vi "main.vi"() -> ()   [LabVIEW 2014]
uses:
  <vilib>/picture/3D Picture Control/Object/Create Object (drawable).vi
  <vilib>/picture/3D Picture Control/Object/Add Object (reference).vi
  <vilib>/Instr/_visa.llb/VISA Configure Serial Port (Instr).vi
  <vilib>/picture/3D Picture Control/NI_3D Picture Control.lvlib
panel:
  out "长度（剩余）":u8
  out "?":u8[](array[numeric])
  in  "选项卡控件":T1
  in  "?":bool
  in  "D":i16
  in  "P":i16
  in  "I":i16
  out "布尔":bool
  out "AcceZ":i32
  out "AcceY":i32
  out "加速度":cluster{dbl, dbl, dbl}(graph)
  out "AcceX":i32
  out "HEANDING":i32
  out "BANK":i32
  out "模块4 2":bool
  out "模块3 2":bool
  out "模块2 2":bool
  out "模块1 2":bool
  out "模块4":bool
  out "模块3":bool
  out "模块2":bool
  out "模块1":bool
  out "PITCH":i32
  in  "停止":bool
  in  "打开":bool caption="stop"
  in  "校验位：":u16(ring) items=["  无校验", "  奇校验", "  偶校验"]
  in  "波特率：":u16(ring)=11 items=["   300", "   600", "   1200", "   2400", "   4800   ", "   9600", "   19200", "   38400", "   43000", "   56000", "   57600", "   115200"]
  in  "通讯口：":u16(ring) items=["   com1", "   com2", "   com3", "   com4", "   com5"]
  out "姿态":cluster{dbl, dbl, dbl}(graph) caption="波形图表"
  in  "上下移动":dbl(slide) scale=-10.0..10.0
  in  "左右移动":dbl(slide) scale=-10.0..10.0
  in  "前后移动":dbl(slide) scale=-10.0..10.0
  in  "缩放":dbl(knob)=2.2771854734286614 scale=0.0..10.0
  out "三维图片":refnum<vi>(3d-picture)
  out "工作指示灯":bool
  # "EVA-MPU6050姿态测试平台"
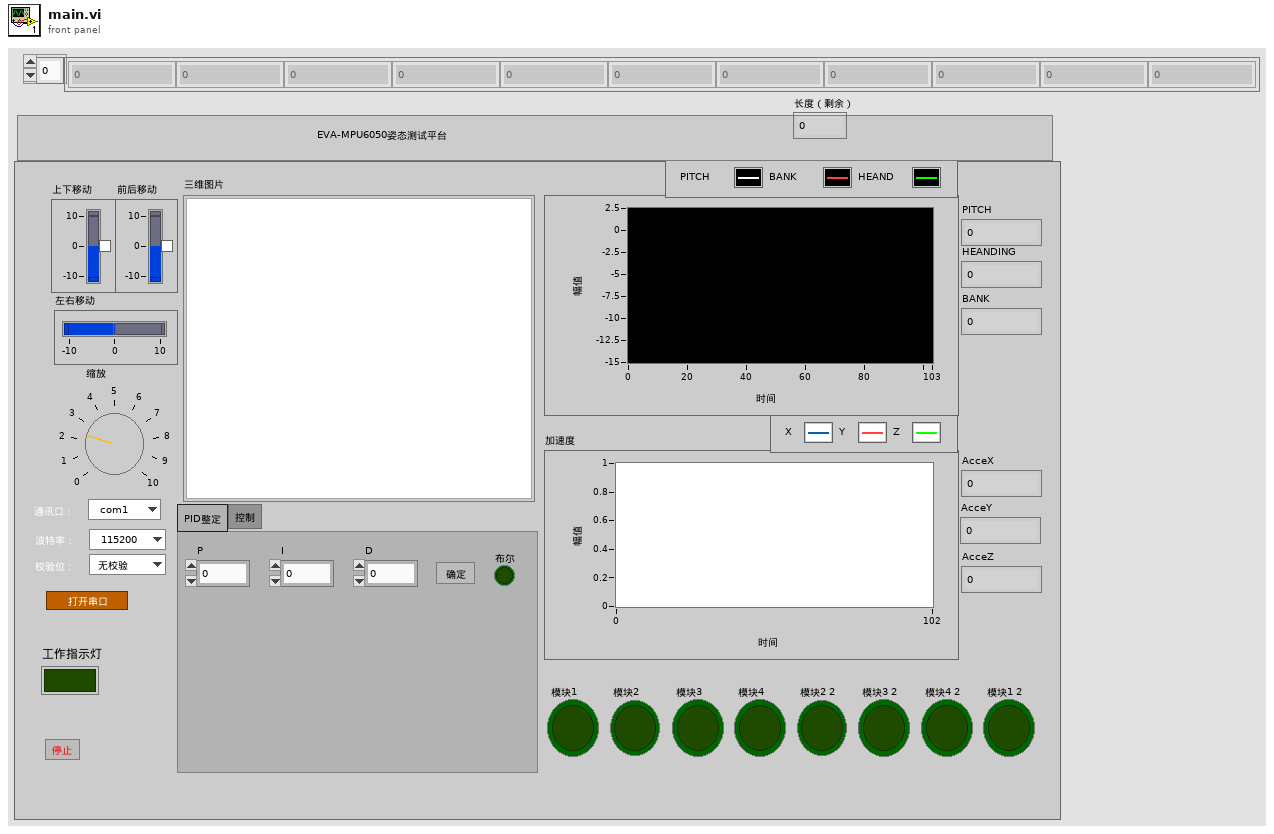
[diagram p1: front panel]
types:
  T1 = typedef "选项卡1.ctl" = enum32{"PID整定", "控制"}
  T2 = cluster{"PITCH":i32, "BANK":i32, "HEANDING":i32, "X":i32, "Y":i32, "Z":i32}
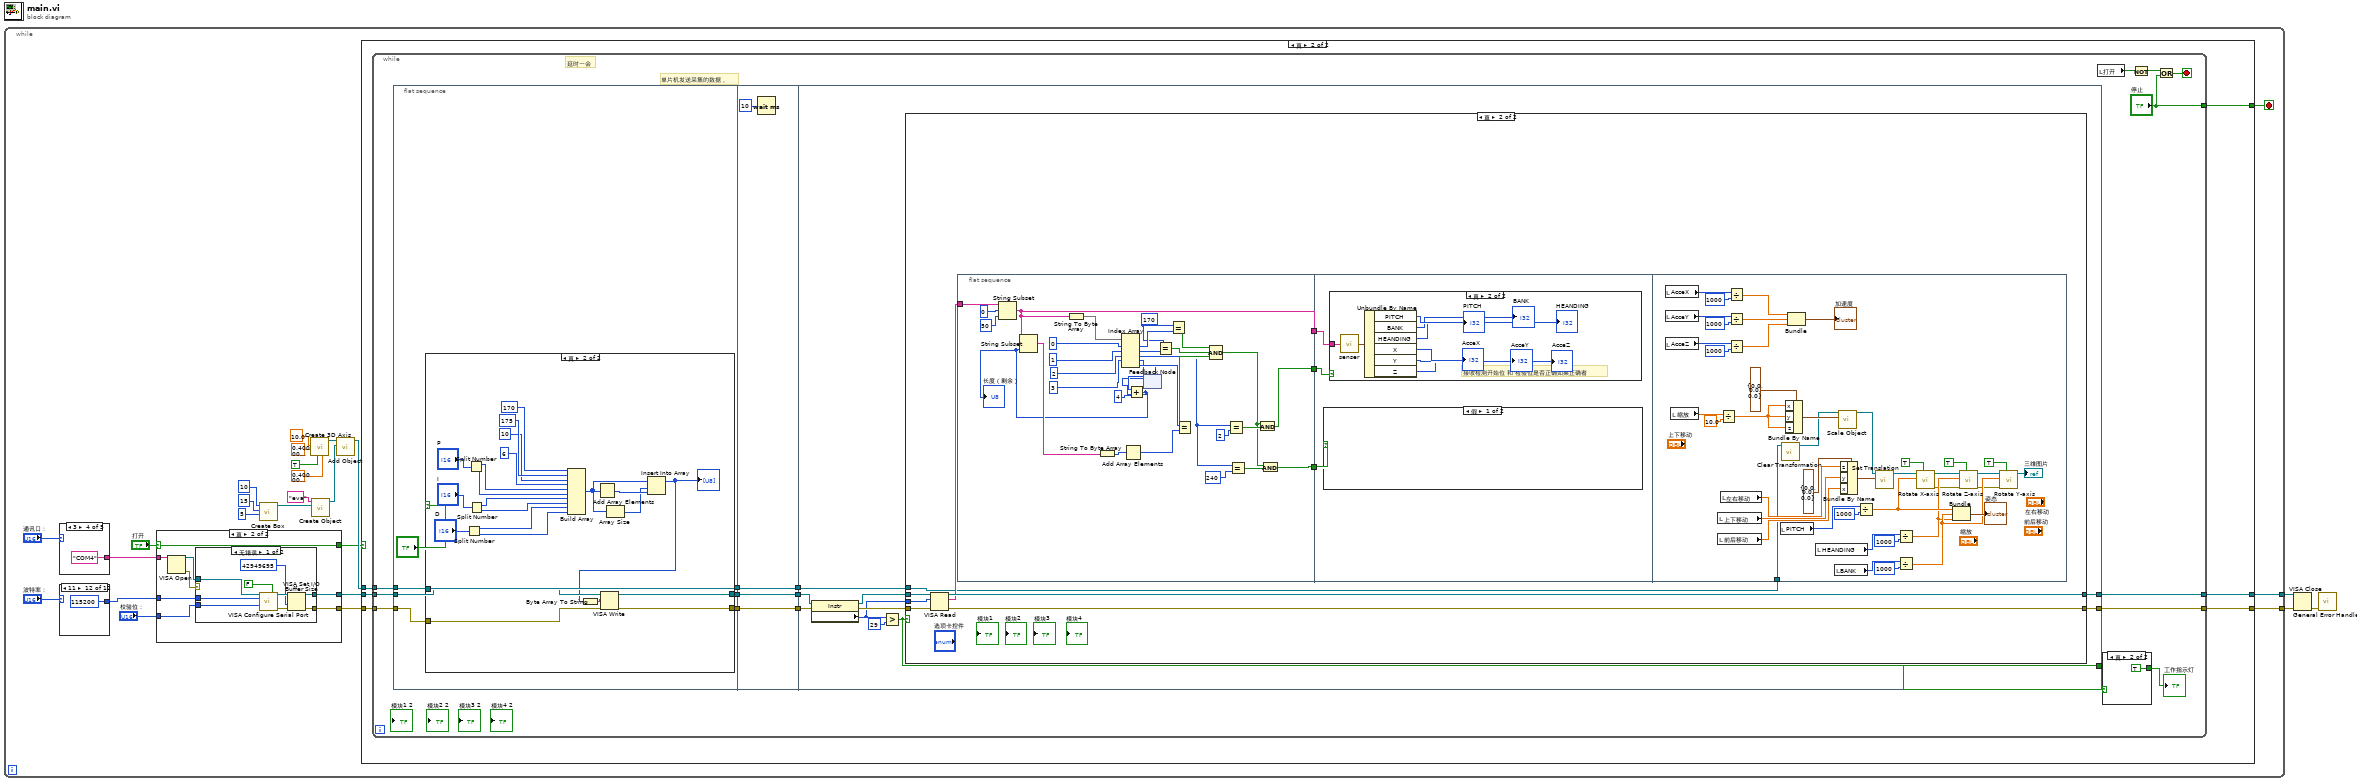
[diagram p0: block diagram]
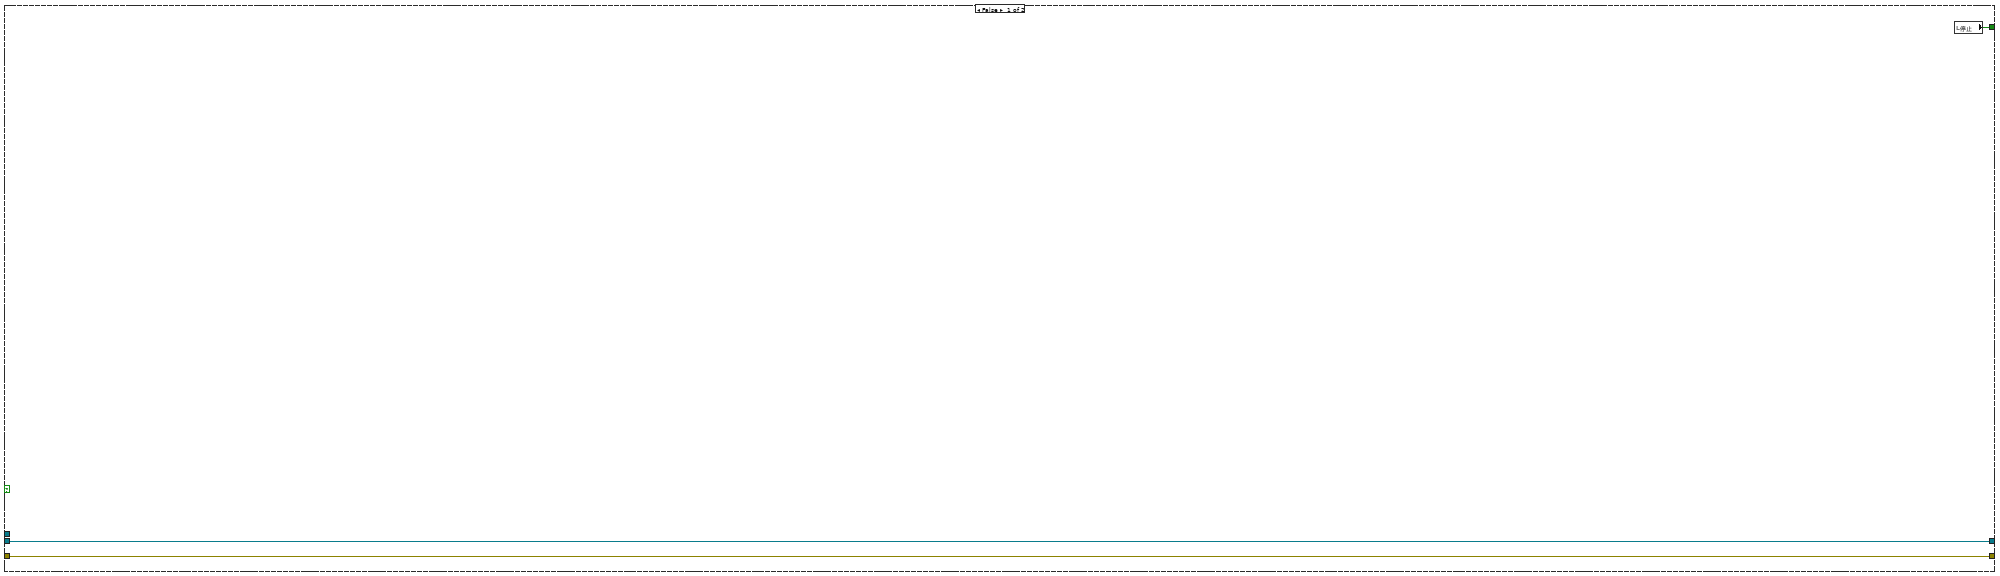
[diagram p2: hidden frame]
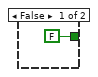
[diagram p3: hidden frame]
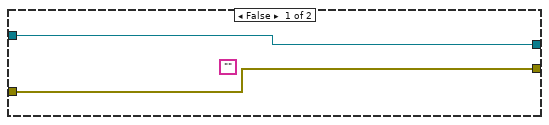
[diagram p4: hidden frame]
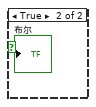
[diagram p6: hidden frame]
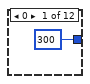
[diagram p8: hidden frame]
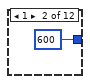
[diagram p9: hidden frame]
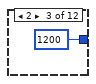
[diagram p10: hidden frame]
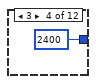
[diagram p11: hidden frame]
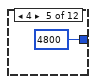
[diagram p12: hidden frame]
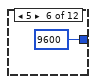
[diagram p13: hidden frame]
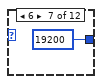
[diagram p14: hidden frame]
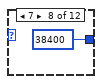
[diagram p15: hidden frame]
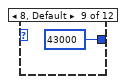
[diagram p16: hidden frame]
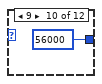
[diagram p17: hidden frame]
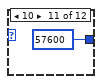
[diagram p18: hidden frame]
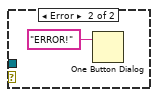
[diagram p20: hidden frame]
diagram:
  n1 = while {
    tunnel: [w26] -> w3
    tunnel: [w25] -> w2
    stop <- w5 stop-if-true
    n2 = case shown="3" "通讯口：" {
      tunnel: ["COM1" "COM2" "COM3" "COM4" "COM5"] -> w9
      frame 0, Default {
      }
      frame 1 {
      }
      frame 2 {
      }
      frame 3 {
      }
      frame 4 {
      }
    }
    n3 = case shown="11" "波特率：" {
      tunnel: [300 600 1200 2400 4800 9600 19200 38400 43000 56000 57600 115200] -> w6
      frame 0 {
      }
      frame 1 {
      }
      frame 2 {
      }
      frame 3 {
      }
      frame 4 {
      }
      frame 5 {
      }
      frame 6 {
      }
      frame 7 {
      }
      frame 8, Default {
      }
      frame 9 {
      }
      frame 10 {
      }
      frame 11 {
      }
    }
    n4 = case shown="真" "打开" {
      selector: "打开" -> [w209 w217]
      tunnel: w6 -> [_ w213]
      tunnel: [w209 w217] -> w4
      tunnel: [_ w211] -> w23
      tunnel: [_ w210] -> w27
      tunnel: w9 -> [_ w216]
      tunnel: "校验位：" -> [_ w212]
      frame False {
      }
      frame True {
        n5 = VISA Open(VISA resource name=w216) -> (VISA resource name=w214:refnum<visa-resource-name>, error out=w215:errorcluster)  [unwired: 4 in]
        n6 = case shown="无错误" w215 {
          tunnel: w214 -> [w226 _]
          tunnel: w213 -> [w225 _]
          tunnel: w212 -> [w224 _]
          tunnel: [w220 _] -> w211
          tunnel: [w221 _] -> w210
          frame No Error {
            n7 = call-poly "VISA Configure Serial Port"("VISA resource name"=w226, "Enable Termination\nChar (T)"=FALSE, "baud rate (9600)"=w225, "parity (0:none)"=w224) -> ("VISA resource name out"=w223:refnum<visa-resource-name>, "error out"=w222:errorcluster)  [unwired: 10 in]
            n8 = VISA Set I/O Buffer Size(VISA resource name=w223, size (4096)=u32 42949695 ("大小(4096)"), error in (no error)=w222) -> (VISA resource name out=w220:refnum<visa-resource-name>, error out=w221:errorcluster)  [unwired: 1 in]
          }
          frame Error {
            n9 = One Button Dialog(message="ERROR!" ("消息")) -> ()  [unwired: 1 in, 1 out]
          }
        }
      }
    }
    n10 = call <vilib>:"Create Box.vi"("Length Z"=5, "Length Y"=15, "Length X"=10) -> ("New Box Refnum"=w18:refnum<vi>)  [unwired: 7 in, 1 out]
    n11 = call <vilib>:"Create 3D Axis.vi"("Character Size"=sgl 0.4, "Axis label?"=TRUE, "Radius"=sgl 0.4, "Length"=sgl 10.0) -> ("New Object Refnum"=w12:refnum<vi>)  [unwired: 6 in, 1 out]
    n12 = call-poly <vilib>:"Create Object.vi"("Geometry"=w18, "Name"="eva") -> ("Scene:New Object"=w17:refnum<vi>)  [unwired: 8 in, 1 out]
    n13 = call-poly <vilib>:"Add Object.vi"("New Object In"=w17, "Scene Object In"=w12) -> ("Scene Object Out"=w24:refnum<vi>)  [unwired: 7 in, 2 out]
    n14 = case shown="真" w4 {
      tunnel: w27 -> [w28 w36]
      tunnel: [w29 w35] -> w26
      tunnel: [w28 w34] -> w25
      tunnel: w24 -> [_ w33]
      tunnel: w23 -> [w29 w32]
      tunnel: [w30 w31] -> w5
      frame False {
        n15 = local read "停止"() -> (w30:bool)
      }
      frame True {
        n16 = while {
          tunnel: w32 -> [w51]
          tunnel: w36 -> [w50]
          tunnel: [w49] -> w35
          tunnel: [w48] -> w34
          tunnel: w33 -> [w45]
          tunnel: ["停止"] -> w31
          stop <- w42 stop-if-true
          # "单片机发送采集的数据，"
          # "延时一会"
          n17 = flat-sequence {
            tunnel: w51 -> [w56]
            tunnel: w50 -> [w57]
            tunnel: w45 -> [w61]
            tunnel: [w61] -> w44
            tunnel: [w59] -> w38
            tunnel: [w58] -> w37
            tunnel: [w89] -> w53
            tunnel: [w88] -> w52
            tunnel: w44 -> [w86]
            tunnel: [w86] -> w43
            tunnel: w38 -> [w89]
            tunnel: w37 -> [w88]
            tunnel: w53 -> [w98]
            tunnel: w52 -> [w97]
            tunnel: [w99] -> w48
            tunnel: [w94] -> w49
            tunnel: [w93] -> w46
            tunnel: w43 -> [w92]
            frame #0 {
              n18 = case shown="真" "?" {
                tunnel: [w63 w82] -> w59
                tunnel: [w62 w81] -> w58
                tunnel: w57 -> [w62 w80]
                tunnel: w56 -> [w63 w79]
                frame False {
                  (unwired) ""
                }
                frame True {
                  n19 = Split Number(x="D") -> (hi(x)=w65:u8, lo(x)=w64:u8)
                  n20 = Split Number(x="P") -> (hi(x)=w71:u8, lo(x)=w70:u8)
                  n21 = Split Number(x="I") -> (hi(x)=w67:u8, lo(x)=w66:u8)
                  n22 = Build Array(u8 170, u8 175, u8 10, u8 6 ("元素"), w71, w70, w67, w66, w65, w64) -> (w75:u8[])
                  n23 = Add Array Elements(numeric array=w75) -> (sum=w76:u8)
                  n24 = Array Size(array=w75) -> (size(s)=w74:i32)
                  n25 = Insert Into Array(array=w75, index=w74, new element=w76) -> (w73:u8[])
                  "?" <- w73
                  n26 = Byte Array To String(unsigned byte array=w73) -> (string=w83:string)
                  n27 = VISA Write(VISA resource name=w79, write buffer=w83, error in (no error)=w80) -> (VISA resource name out=w82:refnum<visa-resource-name>, error out=w81:errorcluster)  [unwired: 1 out]
                }
              }
            }
            frame #1 {
              n28 = Wait (ms)(milliseconds to wait=u32 10 ("等待时间（毫秒）")) -> ()  [unwired: 1 out]
            }
            frame #2 {
              n29 = property class="Instr"(reference=w98, error in=w97) -> (reference out=w96:refnum<visa-resource-name>, error out=w95:errorcluster, "Serial Settings:Number of Bytes at Serial Port"=w91:u32)
              n30 = Greater?(x=w91, y=u32 29) -> (0:w93:bool)
              n31 = case shown="真" w93 {
                tunnel: [w100 w104] -> w99
                tunnel: w96 -> [w101 w111]
                tunnel: w95 -> [w100 w105]
                tunnel: [w101 w110] -> w94
                tunnel: w91 -> [_ w109]
                tunnel: w92 -> [_ w103]
                frame False {
                }
                frame True {
                  n32 = VISA Read(VISA resource name=w111, byte count=w109, error in (no error)=w105) -> (VISA resource name out=w110:refnum<visa-resource-name>, read buffer=w108:string, error out=w104:errorcluster)  [unwired: 1 out]
                  n33 = flat-sequence {
                    tunnel: w108 -> [w134]
                    tunnel: [w133] -> w107
                    tunnel: [w113] -> w106
                    tunnel: [w112] -> w102
                    tunnel: w107 -> [w145]
                    tunnel: w106 -> [w144]
                    tunnel: w102 -> [w143]
                    tunnel: w103 -> [w155]
                    frame #0 {
                      w132 = 170 ("长度（剩余）")
                      n34 = String Subset(string=w134, offset (0)=0 ("长度（剩余）"), length (rest)=50 ("长度（剩余）")) -> (substring=w133:string)
                      n35 = String To Byte Array(string=w133) -> (unsigned byte array=w142:u8[])
                      n36 = feedback #1() -> (w115:u8)  [unwired: 1 in]
                      n37 = Index Array(array=w142, index #1=0 ("长度（剩余）"), index #2=1 ("长度（剩余）"), index #3=2 ("索引"), index #4=3 ("索引"), index #5=w115) -> (element #1=w141:u8, element #2=w131:u8, element #3=w123:u8, element #4=w117:u8, element #5=w125:u8)
                      n38 = Add(x=w117, y=u8 4) -> (x+y=w114:u8)
                      "长度（剩余）" <- w114
                      n39 = String Subset(string=w133, length (rest)=w114) -> (substring=w135:string)  [unwired: 1 in]
                      n40 = String To Byte Array(string=w135) -> (unsigned byte array=w137:u8[])
                      n41 = Add Array Elements(numeric array=w137) -> (sum=w116:u8)
                      n42 = feedback-in #1(w114) -> ()
                      n43 = Equal?(x=w132, y=w131) -> (x = y?=w128:bool)
                      n44 = Equal?(x=w132, y=w141) -> (x = y?=w129:bool)
                      n45 = Equal?(x=w125, y=w116) -> (x = y?=w127:bool)
                      n46 = Compound Arithmetic op=AND(w129, w128, w127) -> (w118:bool)
                      n47 = Equal?(x=w123, y=u8 2) -> (x = y?=w120:bool)
                      n48 = Equal?(x=w123, y=u8 240) -> (x = y?=w119:bool)
                      n49 = And(x=w118, y=w120) -> (x .and. y?=w113:bool)
                      n50 = And(x=w118, y=w119) -> (x .and. y?=w112:bool)
                    }
                    frame #1 {
                      n51 = case shown="假" w143 {
                        selector: w143 -> [_ w146]
                        frame False {
                        }
                        frame True {
                          "布尔" <- w146
                        }
                      }
                      n52 = case shown="真" w144 {
                        tunnel: w145 -> [_ w154]
                        frame False {
                        }
                        frame True {
                          # "接收检测开始位 和 检验位是否正确如果正确者"
                          n53 = call "senser.vi"("read buffer"=w154) -> ("输出簇"=w153:T2)
                          n54 = Unbundle By Name(w153) -> ("PITCH"=→"PITCH":i32, "BANK"=→"BANK":i32, "HEANDING"=→"HEANDING":i32, "X"=→"AcceX":i32, "Y"=→"AcceY":i32, "Z"=→"AcceZ":i32)
                        }
                      }
                    }
                    frame #2 {
                      n55 = local read "AcceX"() -> (w187:i32)
                      n56 = local read "AcceY"() -> (w189:i32)
                      n57 = local read "AcceZ"() -> (w191:i32)
                      n58 = local read "缩放"() -> (w164:dbl)
                      n59 = local read "上下移动"() -> (w166:dbl)
                      n60 = local read "前后移动"() -> (w167:dbl)
                      n61 = Divide(x=w164, y=10.0) -> (x/y=w160:dbl)
                      n62 = local read "左右移动"() -> (w165:dbl)
                      n63 = Divide(x=w187, y=1000) -> (x/y=w193:dbl)
                      n64 = Divide(x=w189, y=1000) -> (x/y=w194:dbl)
                      n65 = Divide(x=w191, y=1000) -> (x/y=w195:dbl)
                      n66 = local read "PITCH"() -> (w181:i32)
                      n67 = call <vilib>:"Clear Transformation.vi"("Object Refnum In"=w155) -> ("Object Refnum Out"=w156:refnum<vi>)  [unwired: 9 in, 1 out]
                      n68 = Bundle By Name(cluster=cluster{"x":dbl, "y":dbl, "z":dbl} {"x"=0.0, "y"=0.0, "z"=0.0}, "x"=w160, "y"=w160, "z"=w160) -> (w158:cluster{"x":dbl, "y":dbl, "z":dbl})
                      n69 = Bundle(w193, w194, w195) -> (→"加速度":cluster{dbl, dbl, dbl})  [unwired: 1 in]
                      n70 = local read "HEANDING"() -> (w185:i32)
                      n71 = local read "BANK"() -> (w180:i32)
                      n72 = call <vilib>:"Scale Object.vi"("Scale"=w158, "Scene.Object In"=w156) -> ("Scene.Object Out"=w157:refnum<vi>)  [unwired: 8 in, 1 out]
                      n73 = Bundle By Name(cluster=cluster{"x":dbl, "y":dbl, "z":dbl} {"x"=0.0, "y"=0.0, "z"=0.0}, "z"=w165, "y"=w166, "x"=w167) -> (w161:cluster{"x":dbl, "y":dbl, "z":dbl})
                      n74 = Divide(x=w181, y=1000) -> (x/y=w182:dbl)
                      n75 = call <vilib>:"Set Translation.vi"("Translation"=w161, "Scene Object"=w157) -> ("Translated Object"=w170:refnum<vi>)  [unwired: 8 in, 1 out]
                      n76 = Divide(x=w185, y=1000) -> (x/y=w179:dbl)
                      n77 = Divide(x=w180, y=1000) -> (x/y=w183:dbl)
                      n78 = call <vilib>:"Rotate X-axis.vi"("Relative?"=TRUE, "angle"=w182, "Scene Object In"=w170) -> ("error out"=w171:errorcluster, "Scene Object Out"=w172:refnum<vi>)  [unwired: 7 in]
                      n79 = Bundle(w182, w183, w179) -> (→"姿态":cluster{dbl, dbl, dbl})  [unwired: 1 in]
                      n80 = call <vilib>:"Rotate Z-axis.vi"("Relative?"=TRUE, "error in (no error)"=w171, "angle"=w179, "Scene Object In"=w172) -> ("error out"=w175:errorcluster, "Scene Object Out"=w176:refnum<vi>)  [unwired: 6 in]
                      n81 = call <vilib>:"Rotate Y-axis.vi"("Relative?"=TRUE, "error in (no error)"=w175, "angle"=w183, "Scene Object In"=w176) -> ("Scene Object Out"=→"三维图片":refnum<vi>)  [unwired: 6 in, 1 out]
                    }
                  }
                }
              }
            }
          }
          n82 = local read "打开"() -> (w40:bool)
          n83 = case shown="真" w46 {
            tunnel: [FALSE ("工作指示灯") TRUE ("工作指示灯")] -> w47
            frame False {
            }
            frame True {
            }
          }
          "工作指示灯" <- w47
          n84 = Not(x=w40) -> (.not. x?=w41:bool)
          n85 = Or(x=w41, y="停止") -> (x .or. y?=w42:bool)
        }
      }
    }
  }
  n86 = VISA Close(VISA resource name=w3, error in (no error)=w2) -> (error out=w1:errorcluster)
  n87 = call <vilib>:"General Error Handler.vi"("error in (no error)"=w1) -> ()  [unwired: 10 in, 5 out]
